vi "Test Init and Close.vi"(8 "error in":errorcluster) -> (0 "error out":errorcluster)   [LabVIEW 2016, in "UT_FileHandler.lvlib"]
doc: "Test the initialization and closing (especially the opend file-reference) of the FileHandler object."
uses:
  UT_FileHandler.lvlib
  Source/HSE-Logger/LogLevel.ctl
  Source/HSE-Logger/Handler/FileHandler/FileHandler.lvclass
  <vilib>/addons/_JKI Toolkits/Caraya/classes/Test/Test.lvclass
  Source/HSE-Logger/hse-logger.lvlib
  <vilib>/addons/_JKI Toolkits/Caraya/classes/Assert/Assert.lvclass
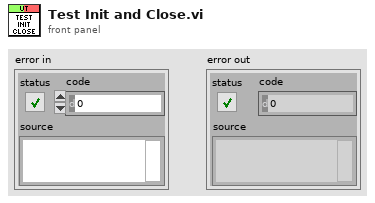
[diagram p1: front panel]
types:
  T1 = typedef "hse-logger.lvlib/LogLevel.ctl" = enum16{"DEBUG", "INFO", "WARNING", "ERROR", "CRITICAL"}
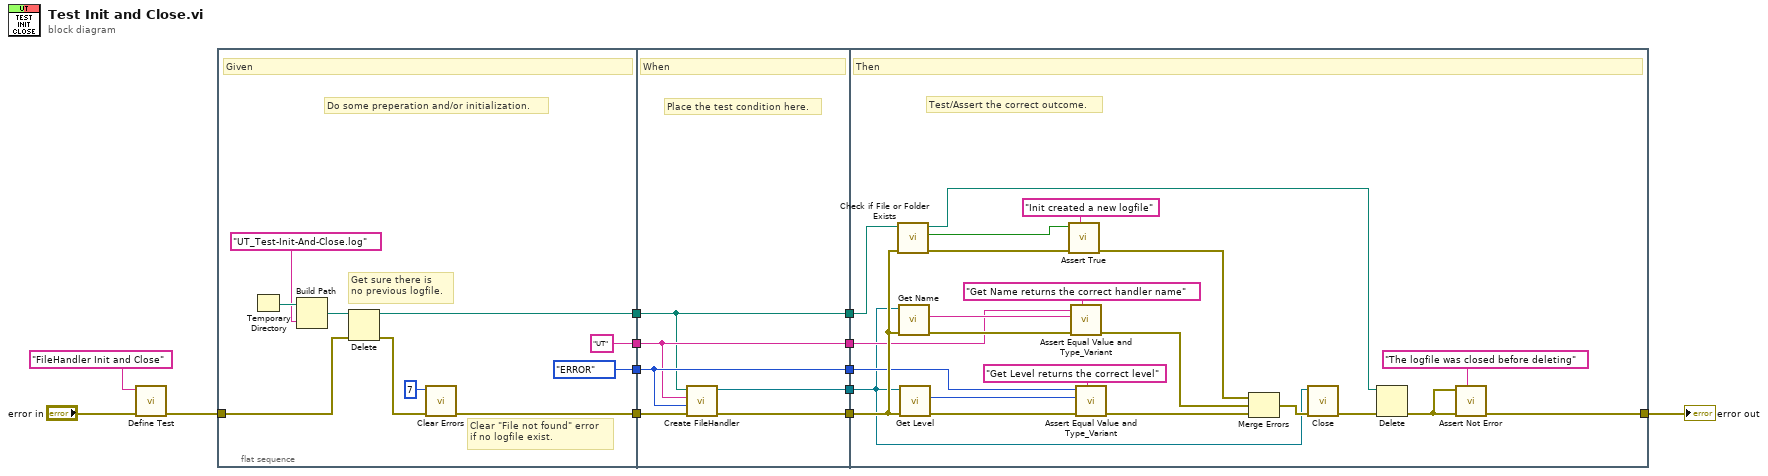
[diagram p0: block diagram]
diagram:
  n1 = call <vilib>:"Define Test.vi"("error in (no error)"="error in", "Label (VI Title)"="FileHandler Init and Close") -> ("error out"=w10:errorcluster)  [unwired: 8 in, 1 out]
  n2 = flat-sequence {
    tunnel: w10 -> [w23]
    tunnel: [w21] -> w13
    tunnel: [LogLevel."ERROR" ("Level")] -> w7
    tunnel: ["UT" ("Name")] -> w6
    tunnel: [w15] -> w5
    tunnel: w13 -> [w29]
    tunnel: [w28] -> w9
    tunnel: w7 -> [w26]
    tunnel: w6 -> [w25]
    tunnel: w5 -> [w24]
    tunnel: [w27] -> w4
    tunnel: [w26] -> w3
    tunnel: [w25] -> w2
    tunnel: [w24] -> w1
    tunnel: [w44] -> w12
    tunnel: w9 -> [w52]
    tunnel: w4 -> [w32]
    tunnel: w3 -> [w40]
    tunnel: w2 -> [w37]
    tunnel: w1 -> [w34]
    frame #0 {
      # "Clear \"File not found\" error\nif no logfile exist."
      # "Get sure there is\nno previous logfile."
      # "Do some preperation and/or initialization."
      # "Given"
      n3 = Temporary Directory() -> (w18:path)
      n4 = Build Path(base path=w18, name or relative path="UT_Test-Init-And-Close.log") -> (appended path=w16:path)
      n5 = Delete(path (use dialog)=w16, error in=w23) -> (deleted path=w15:path, error out=w22:errorcluster)  [unwired: 3 in, 1 out]
      n6 = call <vilib>:"Clear Errors.vi"("error in (no error)"=w22, "specific error code to clear (0: all)"=7) -> ("error out"=w21:errorcluster)  [unwired: 4 in, 1 out]
    }
    frame #1 {
      # "Place the test condition here."
      # "When"
      n7 = call "Create FileHandler.vi"("error in"=w29, "Level"=w26, "Name"=w25, "Filepath"=w24) -> ("error out"=w28:errorcluster, "FileHandler out"=w27:refnum<class "FileHandler.lvclass">)  [unwired: 6 in]
    }
    frame #2 {
      # "Test/Assert the correct outcome."
      # "Then"
      n8 = call <vilib>:"Check if File or Folder Exists.vi"("error in (no error)"=w52, "path"=w34) -> ("error out"=w48:errorcluster, "file or folder exists?"=w33:bool, "dup path"=w30:path)  [unwired: 7 in]
      n9 = call-dynamic "Get Name.vi"("error in"=w52, "Handler in"=w32) -> ("error out"=w49:errorcluster, "Name"=w38:string)  [unwired: 7 in, 1 out]
      n10 = call-dynamic "Get Level.vi"("error in"=w52, "Handler in"=w32) -> ("error out"=w50:errorcluster, "Level"=w41:T1)  [unwired: 7 in, 1 out]
      n11 = call <vilib>:"Assert True.vi"("Label"="Init created a new logfile", "error in (no error)"=w48, "True?"=w33) -> ("error out"=w46:errorcluster)  [unwired: 7 in, 1 out]
      n12 = call <vilib>:"Assert Equal Value and Type_Variant.vi"("Label"="Get Name returns the correct handler name", "error in (no error)"=w49, "Y"=w38, "X"=w37) -> ("error out"=w47:errorcluster)  [unwired: 6 in, 1 out]
      n13 = call <vilib>:"Assert Equal Value and Type_Variant.vi"("Label"="Get Level returns the correct level", "error in (no error)"=w50, "Y"=w41, "X"=w40) -> ("error out"=w51:errorcluster)  [unwired: 6 in, 1 out]
      n14 = Merge Errors(w46, w47, w51) -> (w45:errorcluster)
      n15 = call-dynamic "Close.vi"("error in"=w45, "FileHandler in"=w32) -> ("error out"=w43:errorcluster)  [unwired: 8 in, 1 out]
      n16 = Delete(path (use dialog)=w30, error in=w43) -> (error out=w42:errorcluster)  [unwired: 3 in, 2 out]
      n17 = call <vilib>:"Assert Not Error.vi"("Label"="The logfile was closed before deleting", "error in (no error)"=w42, "Not Error?"=w42) -> ("error out"=w44:errorcluster)  [unwired: 7 in, 1 out]
    }
  }
  "error out" <- w12
